vi "Handle NoTemplatesFound.vi"(8 "error in":errorcluster, 10 "No Templates Found Message":string, 11 "GUI Objects":T1) -> (0 "error out":errorcluster)   [LabVIEW 2022 SP3]
doc: "Initialises or sets up the user-facing front panel (GUI) of the application.\nIncludes:\n1. Setting up the area of the front panel that is displayed to the user\n2. Opening or displaying the front panel"
uses:
  GUI Objects (cluster).ctl
  <vilib>/Utility/miscctls.llb/LVFontTypeDef.ctl
panel:
  # "Development\ncontrols/indicators useful for development and testing, but which are not outputs of the VI"
  # "Input\nInputs to the VI"
  # "Output\nOutputs of the VI"
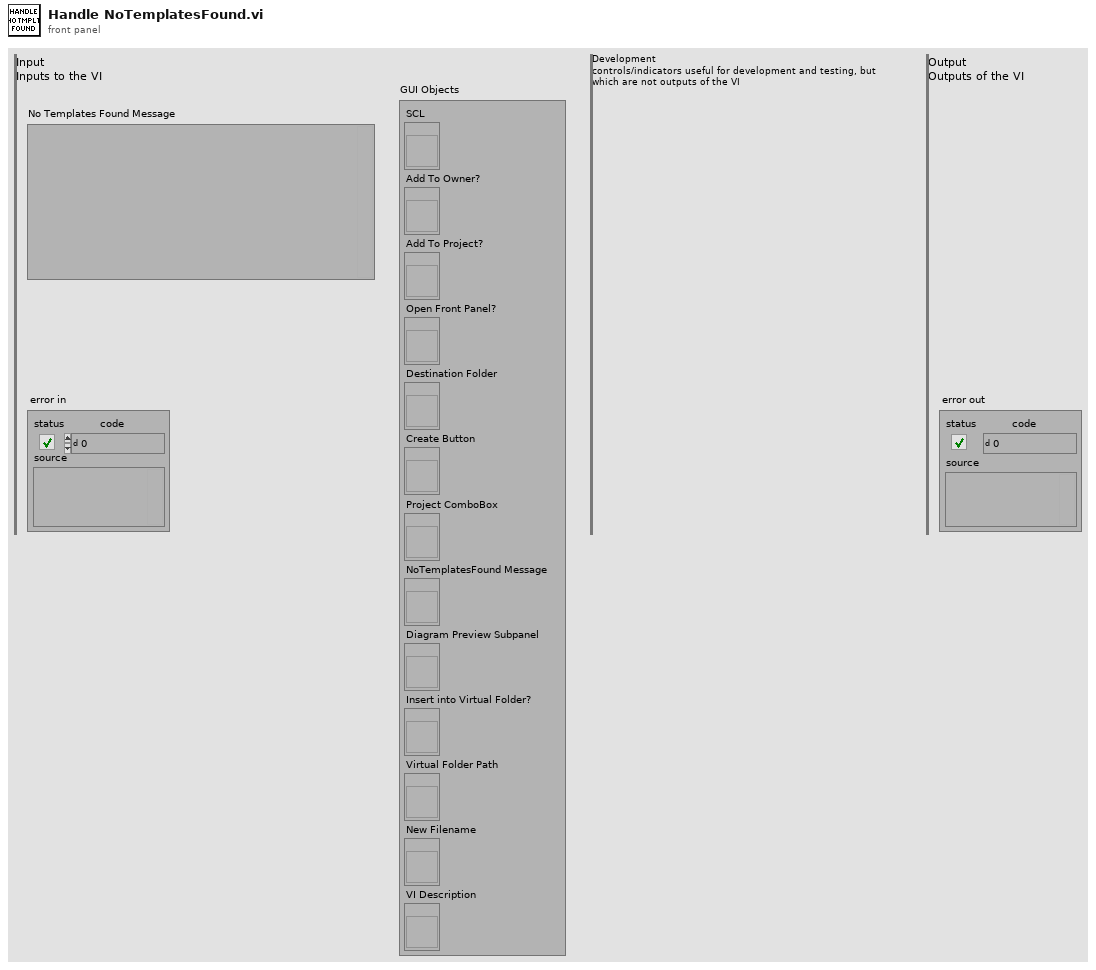
[diagram p1: front panel]
types:
  T1 = typedef "GUI Objects (cluster).ctl" = cluster{"SCL":refnum<vi>, "Add To Owner?":refnum<vi>, "Add To Project?":refnum<vi>, "Open Front Panel?":refnum<vi>, "Destination Folder":refnum<vi>, "Create Button":refnum<vi>, "Project ComboBox":refnum<vi>, "NoTemplatesFound Message":refnum<vi>, "Diagram Preview Subpanel":refnum<vi>, "Insert into Virtual Folder?":refnum<vi>, "Virtual Folder Path":refnum<vi>, "New Filename":refnum<vi>, "VI Description":refnum<vi>}
  T2 = typedef "LVFontTypeDef.ctl" = cluster{"Font Name":string, "Size":u16, "Bold":bool, "Italic":bool, "Underline":bool, "Strikeout":bool, "Color":u32}
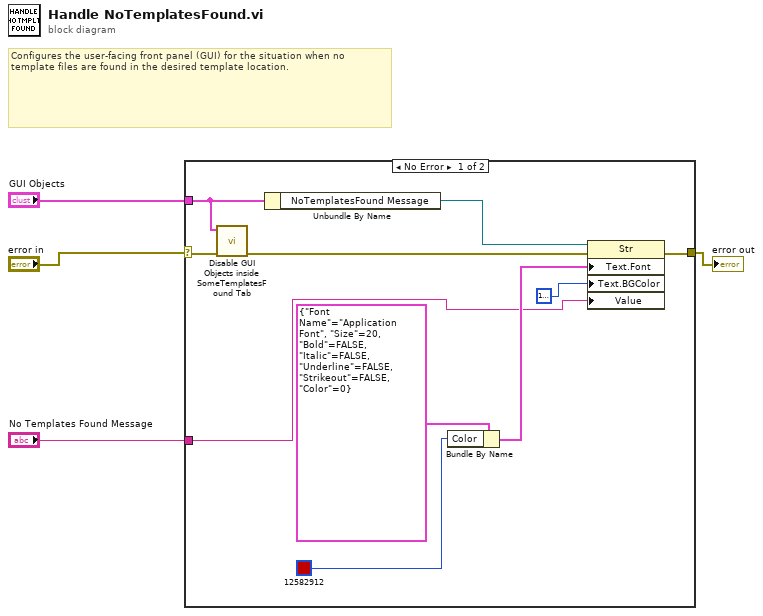
[diagram p0: block diagram]
diagram:
  # "Configures the user-facing front panel (GUI) for the situation when no template files are found in the desired template location."
  n1 = case shown="No Error" "error in" {
    selector: "error in" -> [w14 w15]
    tunnel: [w8 w15] -> w3
    tunnel: "GUI Objects" -> [w6 _]
    tunnel: "No Templates Found Message" -> [w5 _]
    frame No Error {
      n2 = call "Disable GUI Objects inside SomeTemplatesFound Tab.vi"("error in"=w14, "GUI Objects"=w6) -> ("error out"=w7:errorcluster)  [unwired: 9 in]
      n3 = Unbundle By Name(w6) -> ("NoTemplatesFound Message"=w13:refnum<vi>)
      n4 = Bundle By Name(cluster=T2 {"Font Name"="Application Font", "Size"=20, "Bold"=FALSE, "Italic"=FALSE, "Underline"=FALSE, "Strikeout"=FALSE, "Color"=0} ("Text.Font"), "Color"=u32 12582912) -> (w10:T2)
      n5 = property class="Str"(reference=w13, error in=w7, "Text.Font"=w10, "Text.BGColor"=u32 16777216, "Value"=w5) -> (error out=w8:errorcluster)  [unwired: 1 out]
    }
    frame Error {
    }
  }
  "error out" <- w3
